vi "Save method to class.vi"(8 "error in (no error)":errorcluster, 11 "Getter Generator In":refnum<class "Getter Generator.lvclass">) -> (0 "error out":errorcluster, 3 "Getter Generator Out":refnum<class "Getter Generator.lvclass">)   [LabVIEW 2020, in "Method Generation.lvlib" / "Getter Generator.lvclass"]
uses:
  Getter Generator.lvclass
  Getter Generator.lvclass/Getter Generator.ctl
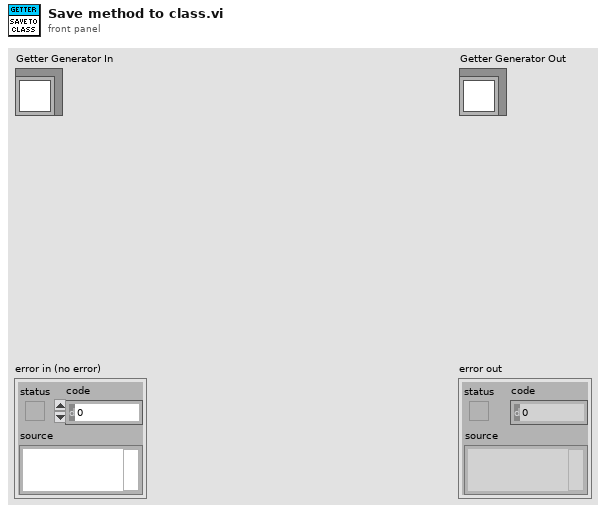
[diagram p1: front panel]
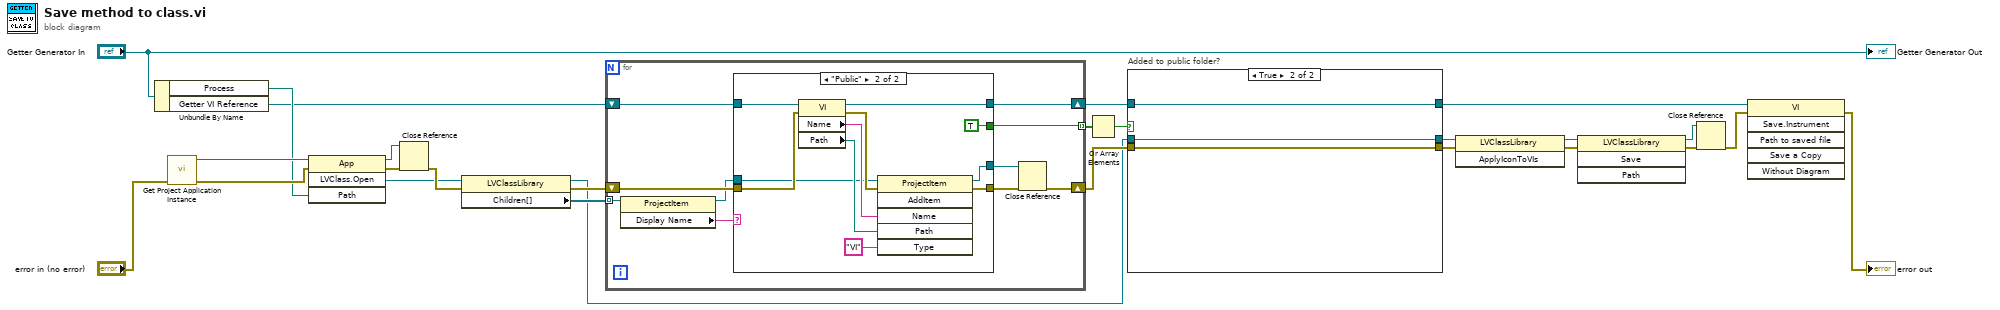
[diagram p0: block diagram]
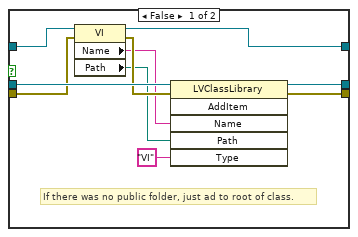
[diagram p2: hidden frame]
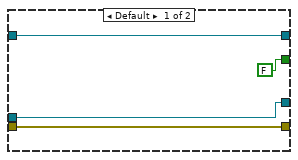
[diagram p3: hidden frame]
diagram:
  n1 = Unbundle By Name("Getter Generator In") -> ("Process"=w23:path, "Getter VI Reference"=w21:refnum<vi>)
  n2 = call "Get Project Application Instance.vi"("error in (no error)"="error in (no error)") -> ("error out"=w24:errorcluster, "Application out"=w25:refnum<vi>)  [unwired: 9 in]
  n3 = invoke class="App" method="LVClass.Open"(reference=w25, error in=w24, "Path"=w23) -> (reference out=w18:refnum<vi>, error out=w20:errorcluster, "LVClass.Open"=w15:refnum<vi>)  [unwired: 1 in, 1 out]
  n4 = Close Reference(reference=w18, error in (no error)=w20) -> (error out=w16:errorcluster)
  n5 = property class="LVClassLibrary"(reference=w15, error in=w16) -> (reference out=w1:refnum<vi>, error out=w9:errorcluster, "Children[]"=w14:refnum<vi>[])
  n6 = for {
    shift-right: [w35] -> w5
    shift-left: w21 -> [w36]
    shift-right: [w29] -> w3
    shift-left: w9 -> [w33]
    tunnel: w14 -> [w30] mode=indexing
    tunnel: [w27] -> w8 mode=indexing
    n7 = property class="ProjectItem"(reference=w30) -> (reference out=w31:refnum<vi>, "Display Name"=w32:string)  [unwired: 1 in, 1 out]
    n8 = case shown="\"Public\"" w32 {
      tunnel: w36 -> [w40 w51]
      tunnel: [w40 w48] -> w35
      tunnel: [w39 w44] -> w34
      tunnel: w33 -> [w39 w45]
      tunnel: w31 -> [w38 w43]
      tunnel: [w38 w42] -> w28
      tunnel: [FALSE TRUE] -> w27
      frame Default {
      }
      frame "Public" {
        n9 = property class="VI"(reference=w51, error in=w45) -> (reference out=w48:refnum<vi>, error out=w49:errorcluster, "Name"=w46:string, "Path"=w50:path)
        n10 = invoke class="ProjectItem" method="AddItem"(reference=w43, error in=w49, "Name"=w46, "Path"=w50, "Type"="VI") -> (reference out=w42:refnum<vi>, error out=w44:errorcluster)  [unwired: 1 in, 4 out]
      }
    }
    n11 = Close Reference(reference=w28, error in (no error)=w34) -> (error out=w29:errorcluster)
  }
  n12 = Or Array Elements(Boolean array=w8) -> (logical OR=w7:bool)
  n13 = case "Added to public folder?" shown="True" w7 {
    tunnel: [w52 w64] -> w6
    tunnel: w5 -> [w61 w64]
    tunnel: [w53 w63] -> w4
    tunnel: w3 -> [w58 w63]
    tunnel: w1 -> [w60 w62]
    tunnel: [w54 w62] -> w2
    frame False {
      # "If there was no public folder, just ad to root of class."
      n14 = property class="VI"(reference=w61, error in=w58) -> (reference out=w52:refnum<vi>, error out=w59:errorcluster, "Name"=w57:string, "Path"=w56:path)
      n15 = invoke class="LVClassLibrary" method="AddItem"(reference=w60, error in=w59, "Name"=w57, "Path"=w56, "Type"="VI") -> (reference out=w54:refnum<vi>, error out=w53:errorcluster)  [unwired: 1 in, 4 out]
    }
    frame True {
    }
  }
  n16 = invoke class="LVClassLibrary" method="ApplyIconToVIs"(reference=w2, error in=w4) -> (reference out=w11:refnum<vi>, error out=w10:errorcluster)  [unwired: 1 in, 1 out]
  n17 = invoke class="LVClassLibrary" method="Save"(reference=w11, error in=w10) -> (reference out=w13:refnum<vi>, error out=w12:errorcluster)  [unwired: 2 in, 2 out]
  n18 = Close Reference(reference=w13, error in (no error)=w12) -> (error out=w17:errorcluster)
  n19 = invoke on="Invoke Node" class="VI" method="Save.Instrument"(reference=w6, error in=w17) -> (error out=→"error out":errorcluster)  [unwired: 4 in, 5 out]
  "Getter Generator Out" <- "Getter Generator In"
